vi "Initialize.vi"(8 "error in (no error)":errorcluster, 9 "Requestor":string, 10 "Requestee":string, 11 "Mag Lab Measure Controller in":refnum<class "Mag Lab Measure Controller.lvclass">) -> (0 "error out":errorcluster, 3 "Mag Lab Measure Controller out":refnum<class "Mag Lab Measure Controller.lvclass">)   [LabVIEW 2015, in "Mag Lab Measure Controller.lvclass"]
uses:
  Mag Lab Measure Controller.lvclass
  Mag Lab Root/Mag Lab Root.lvclass/Mag Lab Root.ctl
  Mag Lab Root Messages/Initialize Msg/Initialize Msg.lvclass/Initialize Msg.ctl
  <vilib>/ActorFramework/Message Enqueuer/Message Enqueuer.lvclass/Message Enqueuer.ctl
  <vilib>/ActorFramework/Message Enqueuer/Enqueue.vi
  <vilib>/ActorFramework/Message Priority Queue/Priority Enqueue.vi
  Mag Lab Root Messages/Initialize Msg/Initialize Msg.lvclass
  Compound Measurement/Compound Measurement.lvclass
  Mag Lab Measure Base/Mag Lab Measure Base.lvclass
  Mag Lab Root/Mag Lab Root.lvclass
  Mag Lab Error Handler/Mag Lab Error Handler.lvclass
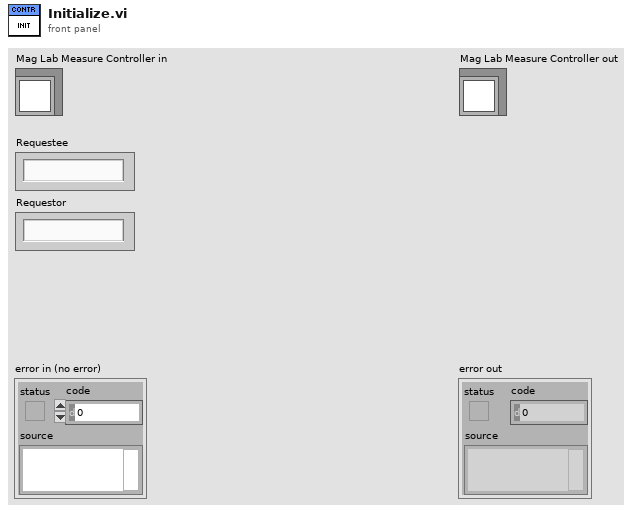
[diagram p1: front panel]
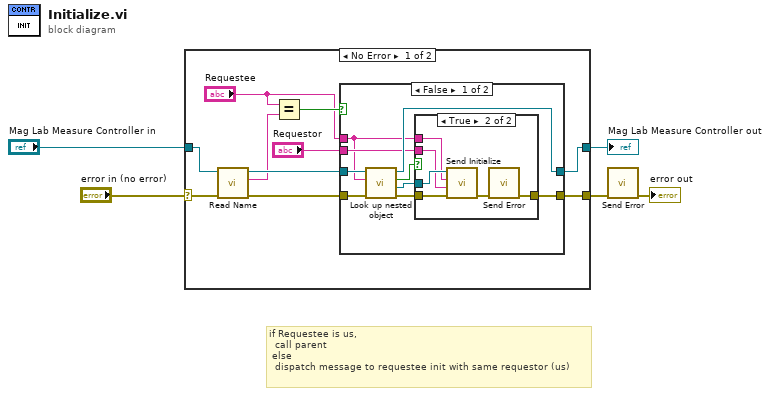
[diagram p0: block diagram]
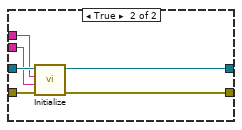
[diagram p3: hidden frame]
diagram:
  # "if Requestee is us, \n\t\tcall parent\n\telse\n\t\tdispatch message to requestee init with same requestor (us)"
  n1 = case shown="No Error" "error in (no error)" {
    selector: "error in (no error)" -> [w12 w39]
    tunnel: [w15 w39] -> w2
    tunnel: [w14 w38] -> w3
    tunnel: "Mag Lab Measure Controller in" -> [w13 w38]
    frame No Error {
      n2 = call "Read Name.vi"("error in (no error)"=w12, "Mag Lab Root in"=w13) -> ("error out"=w8:errorcluster, "Name"=w6:string, "Mag Lab Root out"=w9:refnum<class "Mag Lab Measure Controller.lvclass">)  [unwired: 7 in]
      n3 = Equal?(x="Requestee", y=w6) -> (x = y?=w10:bool)
      n4 = case shown="False" w10 {
        tunnel: [w22 w36] -> w15
        tunnel: [w21 w37] -> w14
        tunnel: "Requestee" -> [w16 w32]
        tunnel: "Requestor" -> [w19 w33]
        tunnel: w9 -> [w17 w35]
        tunnel: w8 -> [w18 w34]
        frame False {
          n5 = call "Look up nested object.vi"("error in (no error)"=w18, "Object name"=w16, "Mag Lab Measure Base in"=w17) -> ("error out"=w23:errorcluster, "Object Queue"=w24:refnum<class "Message Enqueuer.lvclass">, "Found?"=w20:bool, "Mag Lab Measure Base out"=w21:refnum<class "Mag Lab Measure Controller.lvclass">)  [unwired: 5 in]
          n6 = case shown="True" w20 {
            tunnel: w24 -> [_ w31]
            tunnel: w23 -> [w25 w30]
            tunnel: [w25 w26] -> w22
            tunnel: w19 -> [_ w29]
            tunnel: w16 -> [_ w28]
            frame False {
            }
            frame True {
              n7 = call "Send Initialize.vi"("error in (no error)"=w30, "Requestor"=w29, "Requestee"=w28, "Message Enqueuer"=w31) -> ("error out"=w27:errorcluster)  [unwired: 6 in, 1 out]
              n8 = call "Send Error.vi"("error in (no error)"=w27) -> ("error out"=w26:errorcluster)  [unwired: 9 in, 1 out]
            }
          }
        }
        frame True {
          n9 = call-parent "Initialize.vi"("error in (no error)"=w34, "Requestor"=w33, "Requestee"=w32, "Compound Measurement in"=w35) -> ("error out"=w36:errorcluster, "Compound Measurement out"=w37:refnum<class "Mag Lab Measure Controller.lvclass">)  [unwired: 6 in]
        }
      }
    }
    frame Error {
    }
  }
  "Mag Lab Measure Controller out" <- w3
  n10 = call "Send Error.vi"("error in (no error)"=w2) -> ("error out"=→"error out":errorcluster)  [unwired: 9 in, 1 out]
